vi "CurrentRMS.vi"() -> ()   [LabVIEW 2021]
uses:
  <vilib>/DAQmx/read.llb/DAQmx Read (Analog 1D Wfm NChan NSamp).vi
  <vilib>/DAQmx/miscellaneous.llb/DAQmx Fill In Error Info.vi
  <vilib>/measure/madcrms.llb/Averaged DC-RMS for N Chan.vi
  <vilib>/measure/madcrms.llb/Basic Averaged DC-RMS for N Chan.vi
  <vilib>/measure/NI_MAPro.lvlib
panel:
  out "Average":dbl[](graph)
  out "AVG Chart 4":dbl[](graph)
  in  "?":bool
  out "cycle average":dbl[](array[numeric]) format="%.2p"
  out "cycle RMS":dbl[](array[numeric]) format="%.2p"
  out "DC values":dbl[](array[numeric]) format="%.2p"
  out "RMS values":dbl[](array[numeric]) format="%.2p"
  out "Raw Readings":waveform(dbl)[](graph)
  in  "millisecond multiple":u32
  out "DC value waveforms":waveform(dbl)[](array[waveform])
  out "RMS value waveforms":waveform(dbl)[](array[waveform])
  in  "error in":errorcluster
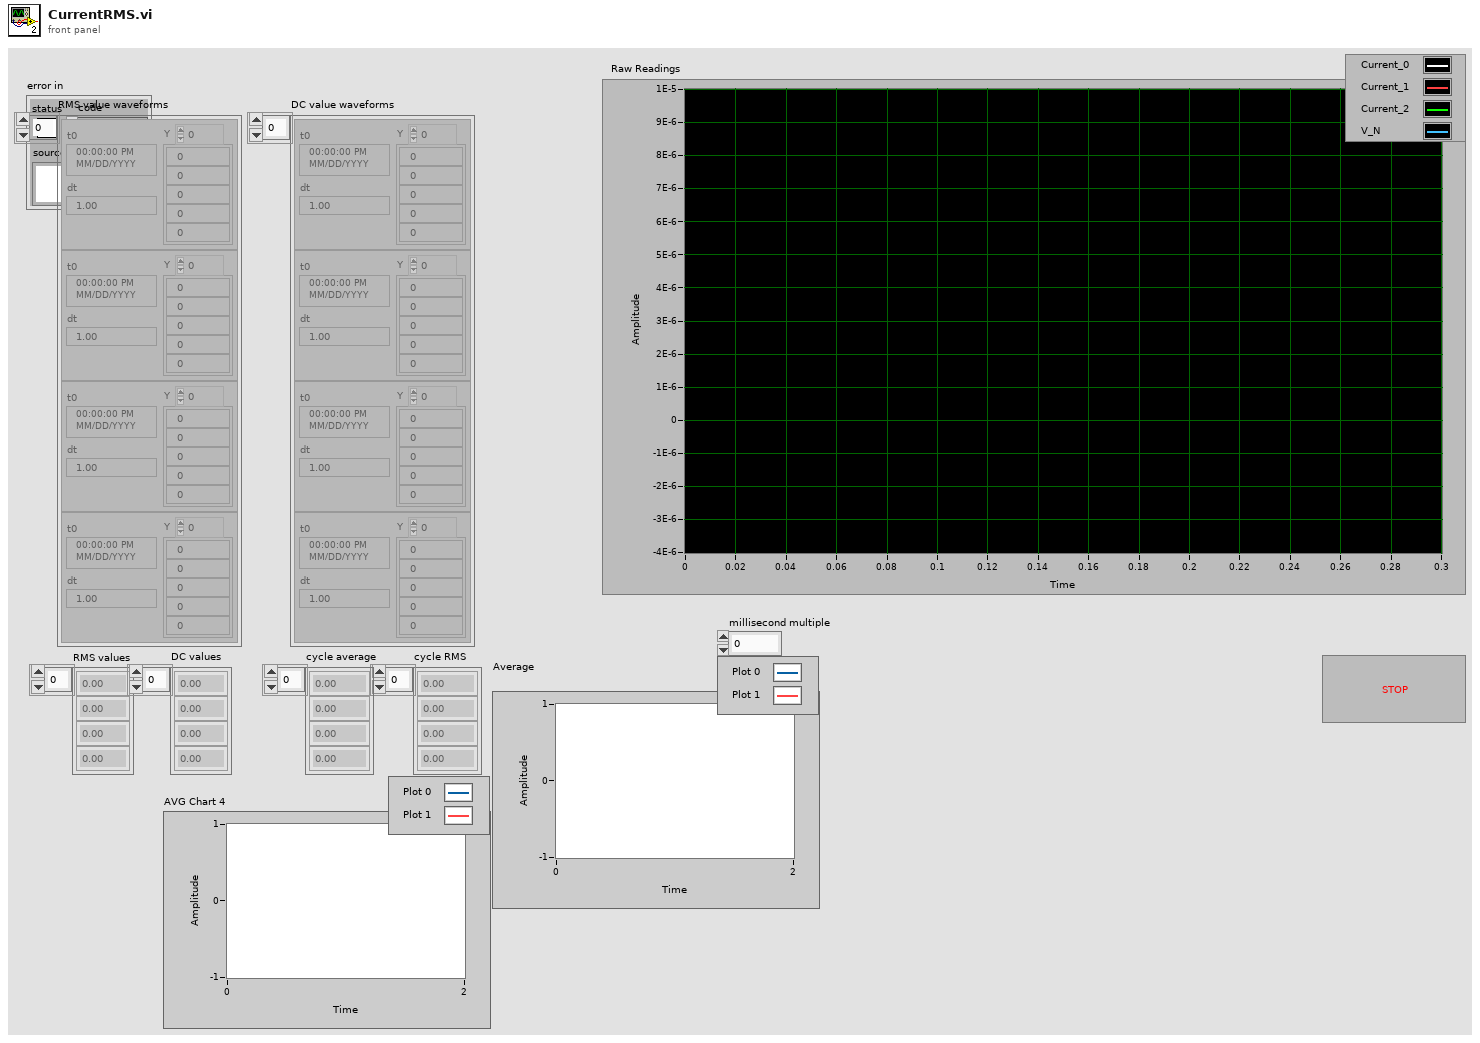
[diagram p1: front panel]
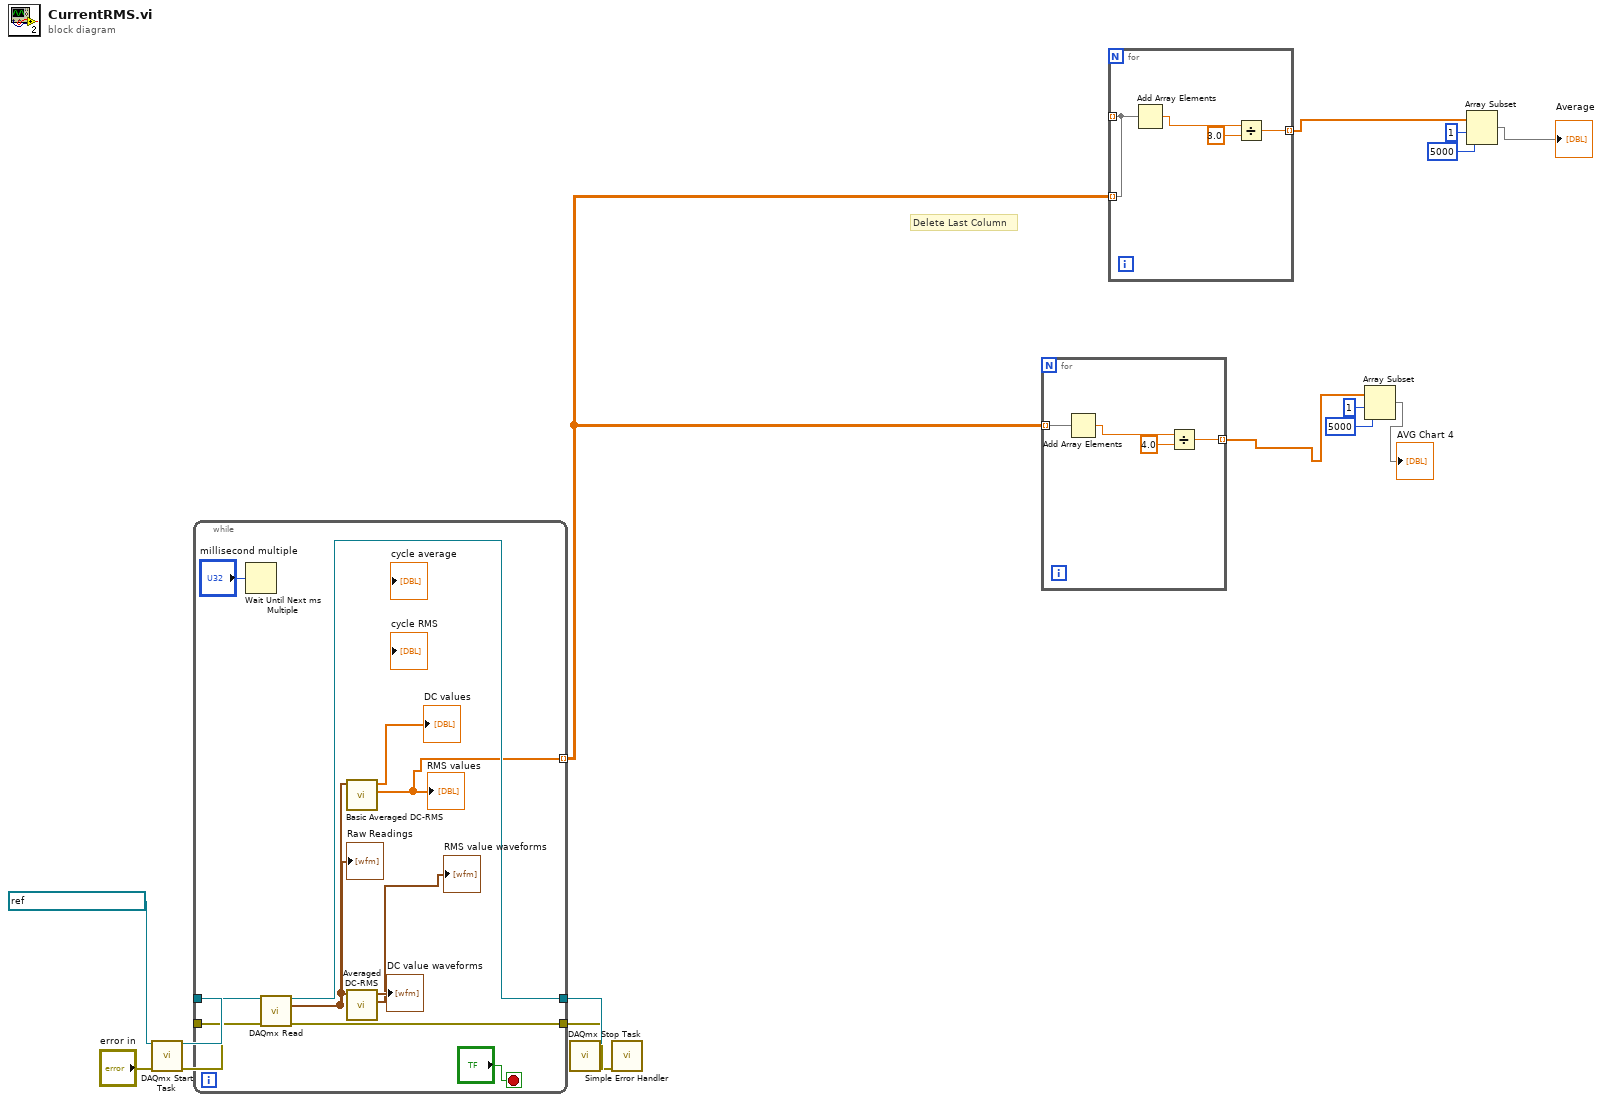
[diagram p0: block diagram]
diagram:
  # "Delete Last Column"
  n1 = call <vilib>:"DAQmx Start Task.vi"("task/channels in"=refnum<k21> "PTS_CAB1k_Currents", "error in"="error in") -> ("task out"=w15:refnum<k21>, "error out"=w13:errorcluster)  [unwired: 12 in]
  n2 = while {
    tunnel: w13 -> [w25]
    tunnel: [w24] -> w12
    tunnel: w15 -> [w27]
    tunnel: [w26] -> w14
    tunnel: [w19] -> w5 mode=indexing
    stop <- "?" stop-if-true
    n3 = Wait Until Next ms Multiple(millisecond multiple="millisecond multiple") -> ()  [unwired: 1 out]
    n4 = call-poly <vilib>:"DAQmx Read.vi"("task/channels in"=w27, "error in"=w25) -> ("task out"=w26:refnum<k21>, "data"=w17:waveform(dbl)[], "error out"=w24:errorcluster)  [unwired: 11 in]
    "Raw Readings" <- w17
    n5 = call-poly <vilib>:"Basic Averaged DC-RMS.vi"("signals in"=w17) -> ("RMS values"=w19:dbl[], "DC values"=→"DC values":dbl[])  [unwired: 7 in, 2 out]
    "RMS values" <- w19
    n6 = call-poly <vilib>:"Averaged DC-RMS.vi"("signals in"=w17) -> ("RMS value waveforms"=→"RMS value waveforms":waveform(dbl)[], "DC value waveforms"=→"DC value waveforms":waveform(dbl)[])  [unwired: 6 in, 3 out]
  }
  n7 = call <vilib>:"DAQmx Stop Task.vi"("task/channels in"=w14, "error in"=w12) -> ("error out"=w11:errorcluster)  [unwired: 12 in, 1 out]
  n8 = call <vilib>:"Simple Error Handler.vi"("error in (no error)"=w11) -> ()  [unwired: 4 in, 5 out]
  n9 = for {
    tunnel: w5 -> [w31] mode=indexing
    tunnel: [w28] -> w7 mode=indexing
    n10 = Add Array Elements(numeric array=w31) -> (sum=w30:dbl)
    n11 = Divide(x=w30, y=4.0) -> (x/y=w28:dbl)
  }
  n12 = for {
    tunnel: [w32] -> _ mode=indexing
    tunnel: [w33] -> w2 mode=indexing
    tunnel: w5 -> [w32] mode=indexing
    n13 = Add Array Elements(numeric array=w32) -> (sum=w35:dbl)
    n14 = Divide(x=w35, y=3.0) -> (x/y=w33:dbl)
  }
  n15 = Array Subset(array=w7, index=1, length=5000) -> (→"AVG Chart 4":dbl[])
  n16 = Array Subset(array=w2, index=1, length=5000) -> (→"Average":dbl[])
